vi "AMC Check Message Queue Status.vi"(7 "error in (no error)":errorcluster, 9 "返回元素？(F)":bool, 10 "Message queue in":T3) -> (0 "error out":errorcluster, 1 "元素":T1[](array[typedef]), 2 "# elements in queue":i32, 3 "Message queue out":T3)   [LabVIEW 2017]
uses:
  Tools/Keyed Array/Tools_KeyedArray KeyedArray.ctl
  subVIs/TypeDefs/amc_Message.ctl
  subVIs/TypeDefs/amc_Message Queue.ctl
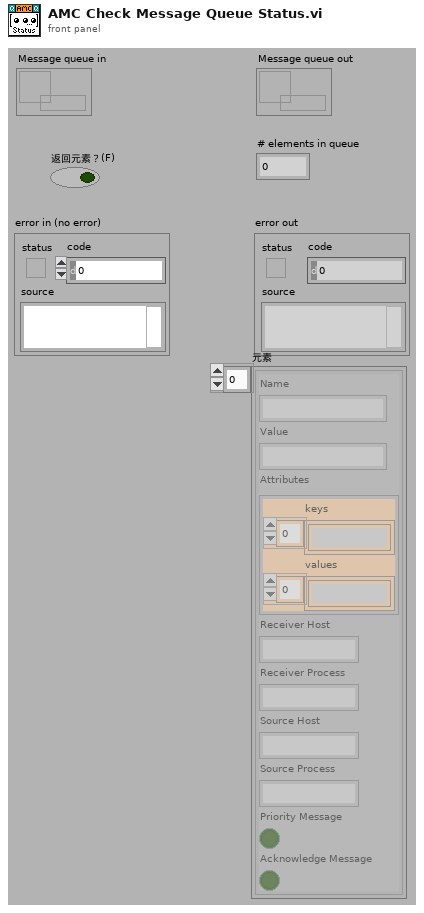
[diagram p1: front panel]
types:
  T1 = typedef "amc_Message.ctl" = cluster{"Name":string, "Value":string, "Attributes":T2, "Receiver Host":string, "Receiver Process":string, "Source Host":string, "Source Process":string, "Priority Message":bool, "Acknowledge Message":bool}
  T2 = typedef "Tools_KeyedArray KeyedArray.ctl" = cluster{"keys":string[], "values":string[]}
  T3 = typedef "amc_Message Queue.ctl" = refnum<queue>
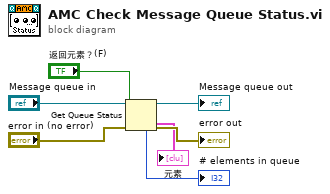
[diagram p0: block diagram]
diagram:
  n1 = Get Queue Status(queue="Message queue in", return elements? (F)="返回元素？(F)", error in (no error)="error in (no error)") -> (queue out=→"Message queue out":T3, error out=→"error out":errorcluster, # elements in queue=→"# elements in queue":i32, elements=→"元素":T1[])  [unwired: 4 out]
